vi "readVoltageSpec.vi"(1 "Channel":i32 min=0 max=15) -> (0 "Voltage":dbl)   [LabVIEW 2011]
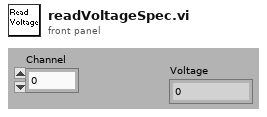
[diagram p1: front panel]
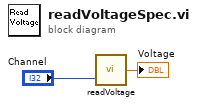
[diagram p0: block diagram]
diagram:
  n1 = call "readVoltage.vi"("Channel Index"="Channel") -> ("Voltage"=→"Voltage":dbl)  [unwired: 1 in]
